vi "HighEnd.vi"() -> ()   [LabVIEW 2016, in "beamline sections.lvlib" / "High energy llb.lvlib"]
uses:
  High energy end/High energy llb.lvlib
  save load/saveloadprev.ctl
  low energy end/Low energy end/Low energy end llb.lvlib
  save load/SaveLoad.lvlib
panel:
  in  "le fc array output":bool[](array[boolean])
  in  "Tab Control":T1(tab)
  out "Analyze magnet readback 2":dbl(graph)=0.8365
  in  "Analyze magnet set":dbl(slide) min=0.0 max=1.6 scale=0.0..1.05
  out "HE Y2 Steerer readback":dbl=2.1859248885760003 format="%#.2g"
  out "He Steerer  X1":dbl=-2.577066196012 format="%#.2g"
  out "He Steerer Y 1":dbl=-0.3914697216320002 format="%#.2g"
  in  "stop":bool
  out "He Quad B readback":dbl=23.541803725959998 format="%#.2g"
  out "He Quad A readback":dbl=12.52186537918 format="%#.2g"
  in  "High Energy Quad A":dbl(slide) scale=17.0..22.0
  in  "High Energy Quad B":dbl(slide) scale=19.0..23.0
  in  "HE Y2 steerer set":dbl(slide)
  in  "High Energy X steerer":dbl(slide) scale=0.5..3.0
  in  "High Energy Y1 steerer":dbl(slide)
  out "Analyze magnet":bool=TRUE
  out "He  1 and 2 Steerer":bool=TRUE
  out "He Quads":bool=TRUE
  in  "Preview-Save-Load":T2
  out "Tank exit ion gauge":cluster{string, string, string, string}
  out "Analyze magnet object":cluster{string, string, string, string}
  out "Analyze magnet readback":dbl=0.8365
  out "He Steerer X1 Voltage +":dbl=3.6657070700000003
  out "He Steerer X1 Voltage -":dbl=6.334092644
  out "He Steerer Y1 Voltage +":dbl=4.932058047
  out "He Steerer Y1 Voltage -":dbl=5.06749495
  out "He Steerer Y2 Voltage +":dbl=4.216001645
  out "He Steerer Y2 Voltage -":dbl=5.783759862
  out "He Steerer X1 Readback Voltage -":dbl=4.638408521444
  out "He Steerer Y1 Readback  +":dbl=6.277195359484
  out "He Steerer Y1 Readback  -":dbl=3.6955313647279997
  out "He Steerer Y2  Readback +":dbl=4.020661418768
  out "He Steerer Y2  Readback -":dbl=6.050261150048
  out "He Steerer X1 Readback Voltage +":dbl=5.03119189986
  in  "HighEnd temp file":path=path "D:/Main Tune Parameters/Temp Configs/HighEnd.txt"
  out "SaveLoad Error":errorcluster
  out "SV error":errorcluster
  # "High Energy End"
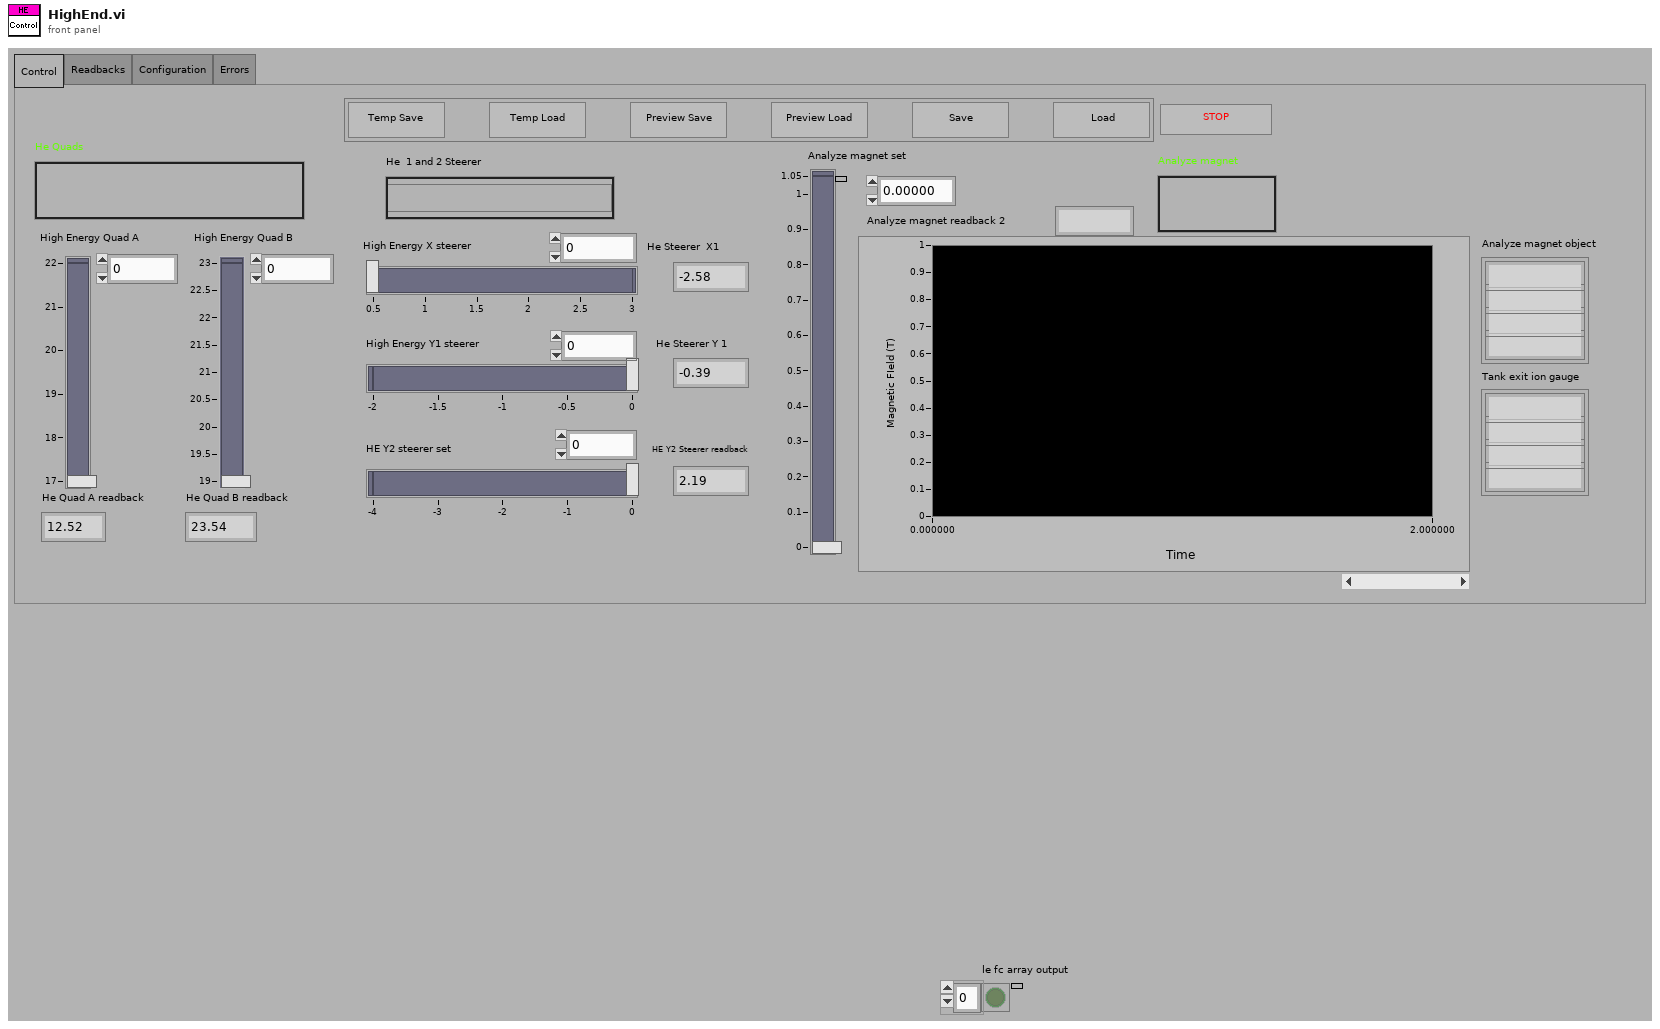
[diagram p1: front panel]
types:
  T1 = enum32{"Control", "Readbacks", "Configuration", "Errors"}
  T2 = typedef "saveloadprev.ctl" = cluster{"Temp Save":bool, "Temp Load":bool, "Save":bool, "Load":bool, "Preview Save":bool, "Preview Load":bool}
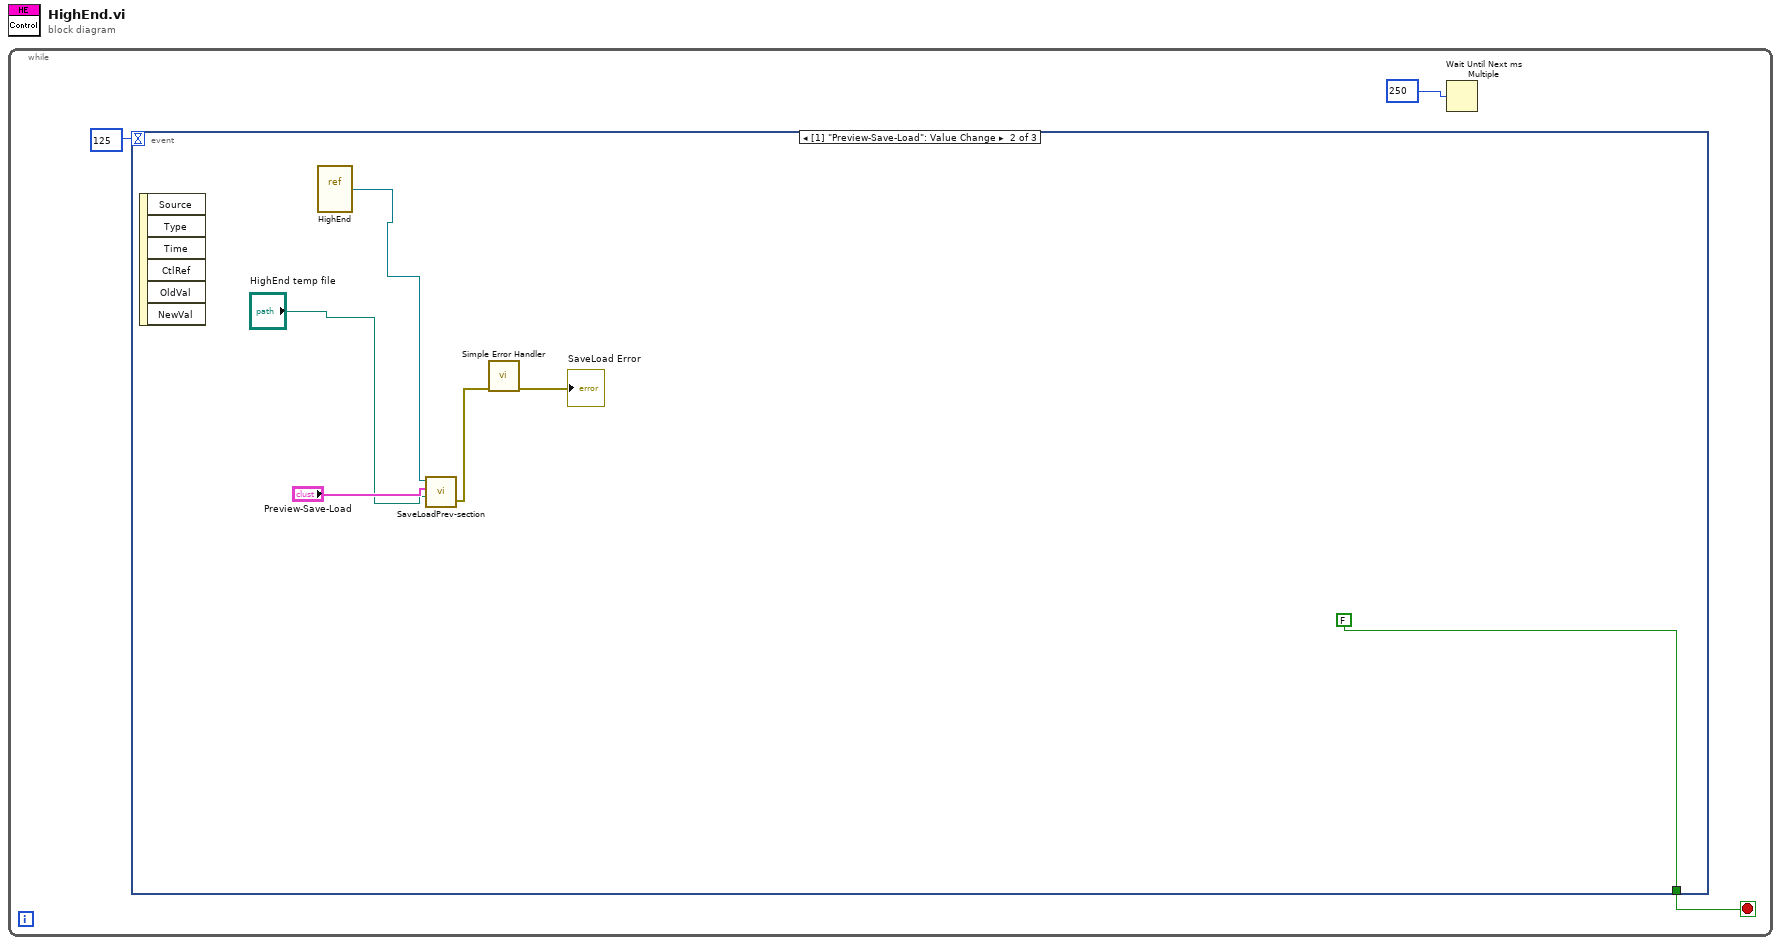
[diagram p0: block diagram]
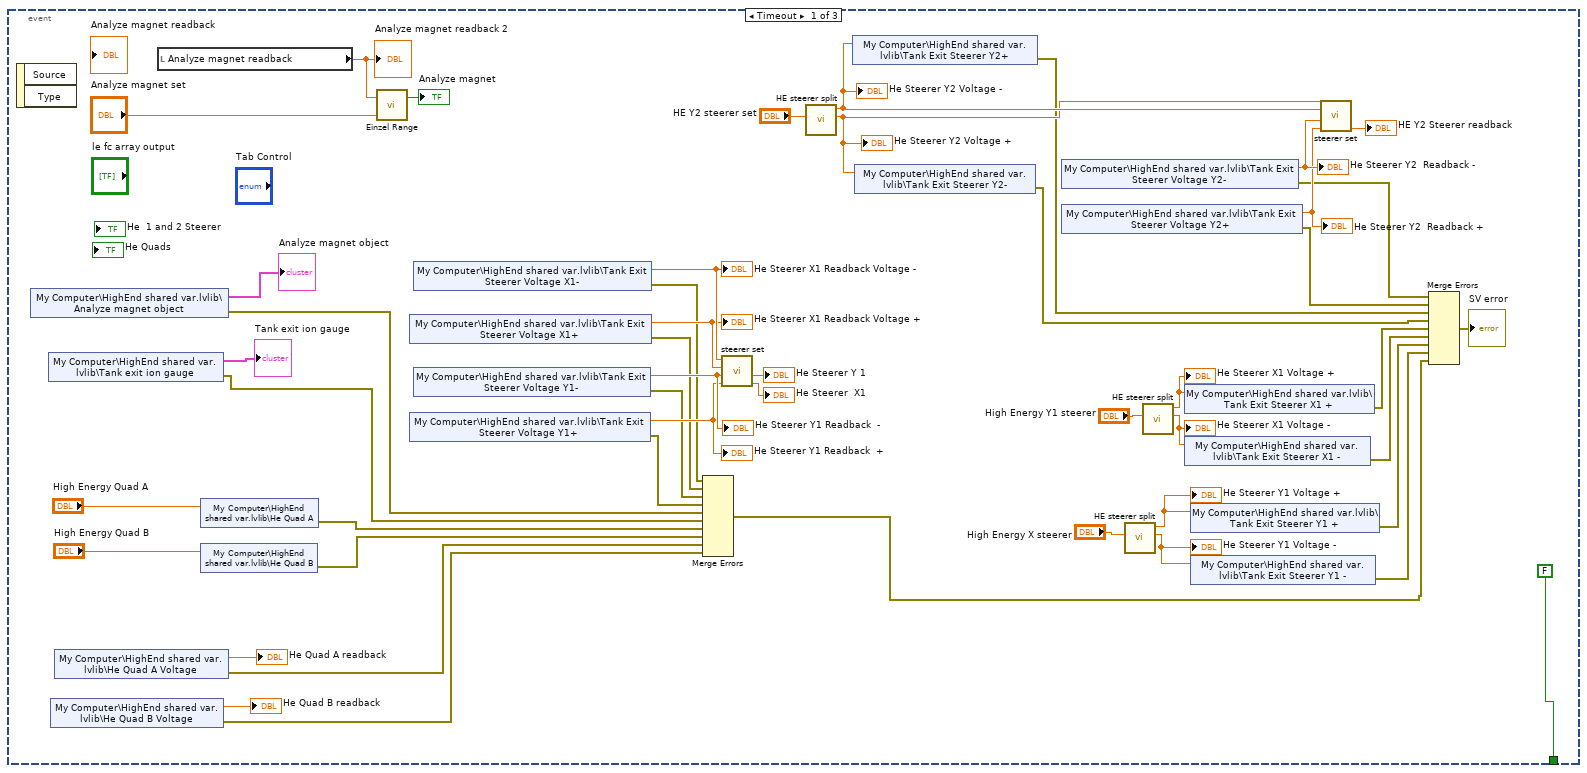
[diagram p2: hidden frame]
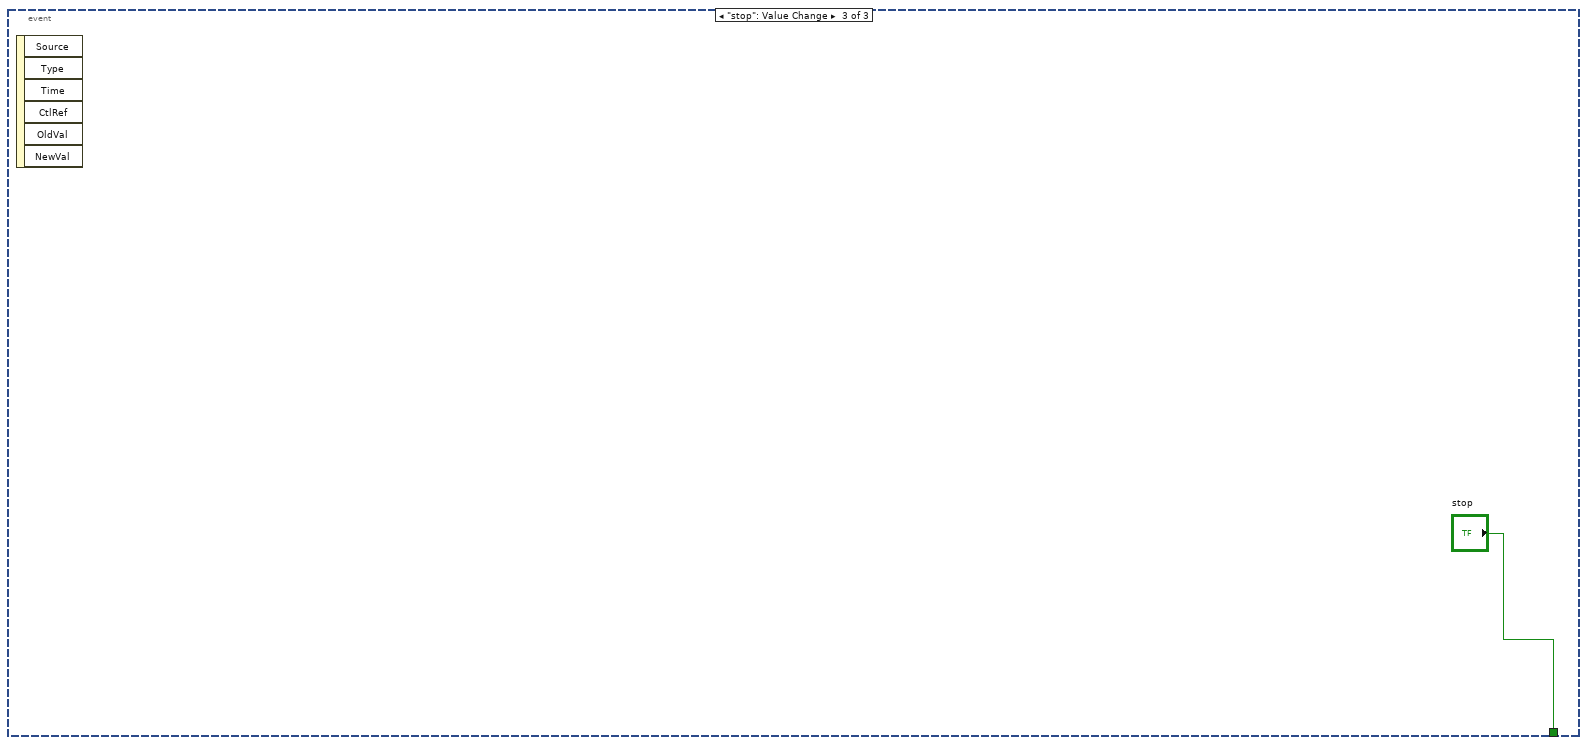
[diagram p3: hidden frame]
diagram:
  n1 = while {
    stop <- w1 stop-if-true
    n2 = event shown="[1] \"Preview-Save-Load\": Value Change" {
      selector: _ -> [_ _ _]
      dyn-events: _ -> [_ _ _]
      timeout: 125 -> [_ _ _]
      tunnel: [FALSE FALSE "stop"] -> w1
      event Timeout {
        n3 = event-data() -> ()  [unwired: 1 in, 2 out]
        n4 = shared-variable "My Computer\\HighEnd shared var.lvlib\\Analyze magnet object"() -> (→"Analyze magnet object":cluster{string, string, string, string}, error out=w19:errorcluster)  [unwired: 1 in]
        n5 = shared-variable "My Computer\\HighEnd shared var.lvlib\\Tank exit ion gauge"() -> (→"Tank exit ion gauge":cluster{string, string, string, string}, error out=w18:errorcluster)  [unwired: 1 in]
        n6 = shared-variable "My Computer\\HighEnd shared var.lvlib\\He Quad B Voltage"() -> (→"He Quad B readback":dbl, error out=w14:errorcluster)  [unwired: 1 in]
        n7 = shared-variable "My Computer\\HighEnd shared var.lvlib\\He Quad A Voltage"() -> (→"He Quad A readback":dbl, error out=w15:errorcluster)  [unwired: 1 in]
        n8 = local read "Analyze magnet readback"() -> (w36:dbl)
        "Analyze magnet readback 2" <- w36
        n9 = shared-variable "My Computer\\HighEnd shared var.lvlib\\He Quad A"("High Energy Quad A") -> (error out=w17:errorcluster)  [unwired: 1 in]
        n10 = shared-variable "My Computer\\HighEnd shared var.lvlib\\He Quad B"("High Energy Quad B") -> (error out=w16:errorcluster)  [unwired: 1 in]
        n11 = call "Einzel Range.vi"("Inj image Readback"="Analyze magnet set", "Inj image Einzel Set"=w36) -> ("Einzel  Range"=→"Analyze magnet":bool)  [unwired: 1 out]
        n12 = shared-variable "My Computer\\HighEnd shared var.lvlib\\Tank Exit Steerer Voltage X1+"() -> (w26:dbl, error out=w22:errorcluster)  [unwired: 1 in]
        "He Steerer X1 Readback Voltage +" <- w26
        n13 = shared-variable "My Computer\\HighEnd shared var.lvlib\\Tank Exit Steerer Voltage Y1+"() -> (w25:dbl, error out=w20:errorcluster)  [unwired: 1 in]
        "He Steerer Y1 Readback  +" <- w25
        n14 = shared-variable "My Computer\\HighEnd shared var.lvlib\\Tank Exit Steerer Voltage X1-"() -> (w27:dbl, error out=w23:errorcluster)  [unwired: 1 in]
        "He Steerer X1 Readback Voltage -" <- w27
        n15 = shared-variable "My Computer\\HighEnd shared var.lvlib\\Tank Exit Steerer Voltage Y1-"() -> (w29:dbl, error out=w21:errorcluster)  [unwired: 1 in]
        "He Steerer Y1 Readback  -" <- w29
        n16 = Merge Errors(w23, w22, w21, w20, w19, w18, w17, w16, w15, w14) -> (w5:errorcluster)
        n17 = call "steerer set.vi"("Injector image X  -"=w27, "Injector image X +"=w26, "Injector image Y  -"=w29, "Injector image Y +"=w25) -> ("Steerer X"=→"He Steerer Y 1":dbl, "Steerer Y"=→"He Steerer  X1":dbl)  [unwired: 4 out]
        n18 = call "HE steerer split.vi"("Steerer in"="HE Y2 steerer set") -> ("Steerer +"=w42:dbl, "Steerer -"=w41:dbl)  [unwired: 7 out]
        "He Steerer Y2 Voltage +" <- w41
        "He Steerer Y2 Voltage -" <- w42
        n19 = shared-variable "My Computer\\HighEnd shared var.lvlib\\Tank Exit Steerer Y2+"(w42) -> (error out=w13:errorcluster)  [unwired: 1 in]
        n20 = shared-variable "My Computer\\HighEnd shared var.lvlib\\Tank Exit Steerer Y2-"(w41) -> (error out=w12:errorcluster)  [unwired: 1 in]
        n21 = shared-variable "My Computer\\HighEnd shared var.lvlib\\Tank Exit Steerer Voltage Y2-"() -> (w45:dbl, error out=w11:errorcluster)  [unwired: 1 in]
        "He Steerer Y2  Readback -" <- w45
        n22 = shared-variable "My Computer\\HighEnd shared var.lvlib\\Tank Exit Steerer Voltage Y2+"() -> (w44:dbl, error out=w10:errorcluster)  [unwired: 1 in]
        "He Steerer Y2  Readback +" <- w44
        n23 = call "HE steerer split.vi"("Steerer in"="High Energy X steerer") -> ("Steerer +"=w30:dbl, "Steerer -"=w31:dbl)  [unwired: 7 out]
        "He Steerer Y1 Voltage +" <- w30
        "He Steerer Y1 Voltage -" <- w31
        n24 = call "HE steerer split.vi"("Steerer in"="High Energy Y1 steerer") -> ("Steerer +"=w33:dbl, "Steerer -"=w34:dbl)  [unwired: 7 out]
        "He Steerer X1 Voltage +" <- w33
        "He Steerer X1 Voltage -" <- w34
        n25 = shared-variable "My Computer\\HighEnd shared var.lvlib\\Tank Exit Steerer X1 +"(w33) -> (error out=w9:errorcluster)  [unwired: 1 in]
        n26 = shared-variable "My Computer\\HighEnd shared var.lvlib\\Tank Exit Steerer X1 -"(w34) -> (error out=w8:errorcluster)  [unwired: 1 in]
        n27 = shared-variable "My Computer\\HighEnd shared var.lvlib\\Tank Exit Steerer Y1 +"(w30) -> (error out=w7:errorcluster)  [unwired: 1 in]
        n28 = shared-variable "My Computer\\HighEnd shared var.lvlib\\Tank Exit Steerer Y1 -"(w31) -> (error out=w6:errorcluster)  [unwired: 1 in]
        n29 = call "steerer set.vi"("Injector image X  -"=w41, "Injector image X +"=w42, "Injector image Y  -"=w45, "Injector image Y +"=w44) -> ("Steerer Y"=→"HE Y2 Steerer readback":dbl)  [unwired: 5 out]
        n30 = Merge Errors(w11, w10, w13, w12, w9, w8, w7, w6, w5) -> (→"SV error":errorcluster)
      }
      event Value Change {
        n31 = event-data() -> ()  [unwired: 1 in, 6 out]
        n32 = vi-ref "HighEnd.vi"() -> (w54:refnum<vi>)
        n33 = call "SaveLoadPrev-section.vi"("file path (use dialog)"="HighEnd temp file", "Cluster 2"="Preview-Save-Load", "VI Refnum"=w54) -> ("error out"=w53:errorcluster)  [unwired: 2 in]
        n34 = call <vilib>:"Simple Error Handler.vi"("error in (no error)"=w53) -> ("error out"=→"SaveLoad Error":errorcluster)  [unwired: 4 in, 4 out]
      }
      event "stop": Value Change {
        n35 = event-data() -> ()  [unwired: 1 in, 6 out]
      }
    }
    n36 = Wait Until Next ms Multiple(millisecond multiple=u32 250) -> ()  [unwired: 1 out]
  }
